vi "TCPIP_Server.vi"(9 "Message from Client":refnum<queue>, 10 "Data to TCPIP":refnum<queue>) -> ()   [LabVIEW 2018]
uses:
  TCP Multiple Connections State.ctl
  TCP Multiple Connections Data.ctl
panel:
  out "# of Connections":i32
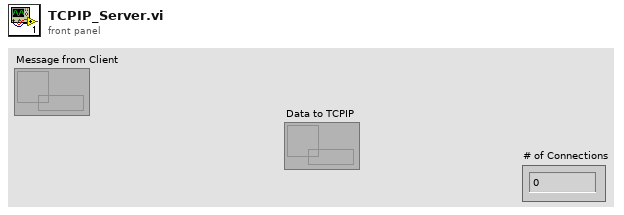
[diagram p1: front panel]
types:
  T1 = typedef "TCP Multiple Connections Data.ctl" = cluster{"Clients":refnum<k5>[], "Listener":refnum<k5>}
  T2 = typedef "TCP Multiple Connections State.ctl" = enum16{"Initialize", "Status Check", "Send Data", "Stop"}
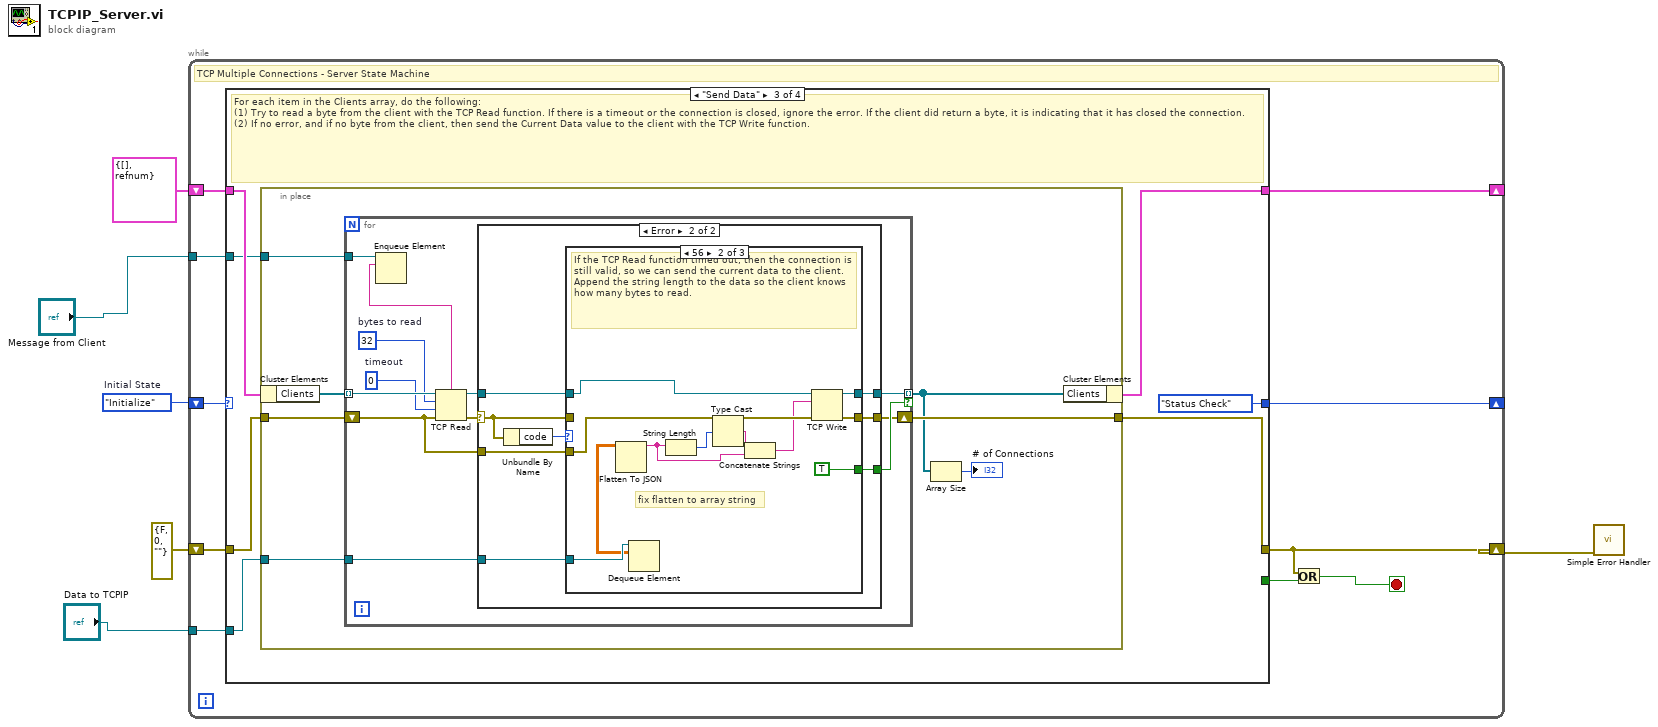
[diagram p0: block diagram]
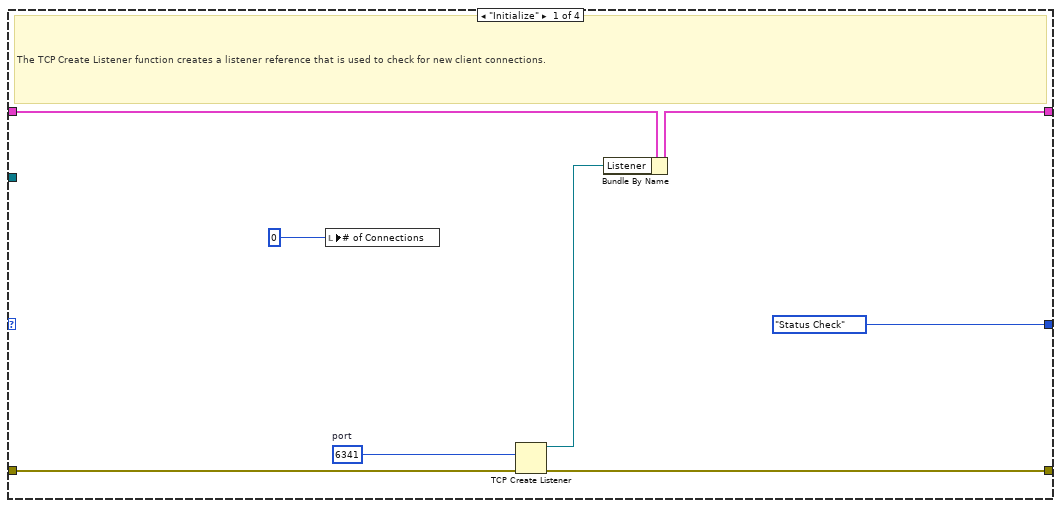
[diagram p2: hidden frame]
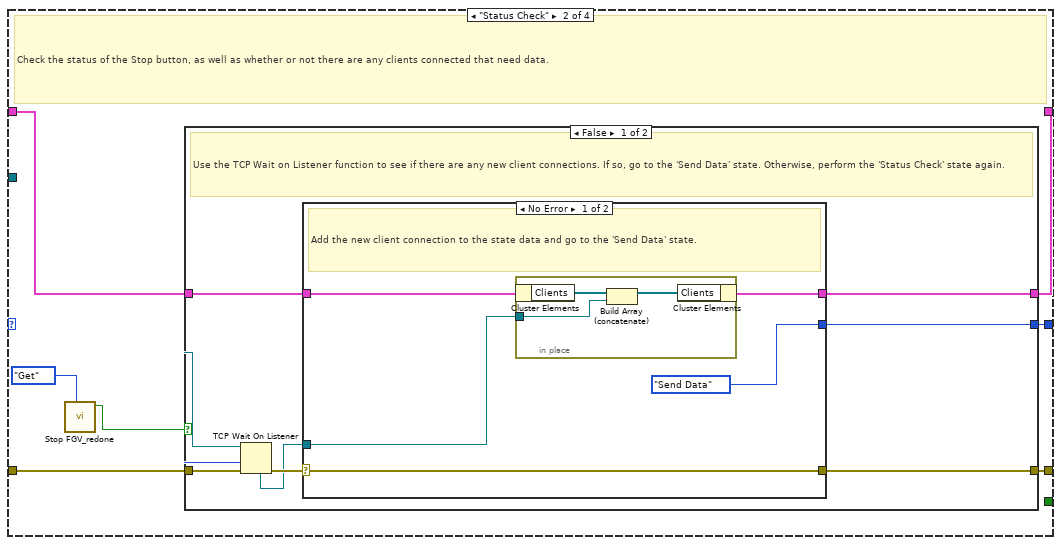
[diagram p3: hidden frame]
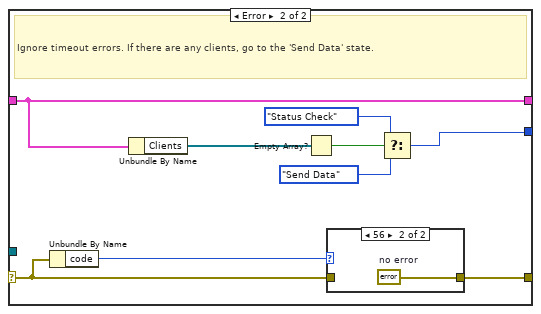
[diagram p4: hidden frame]
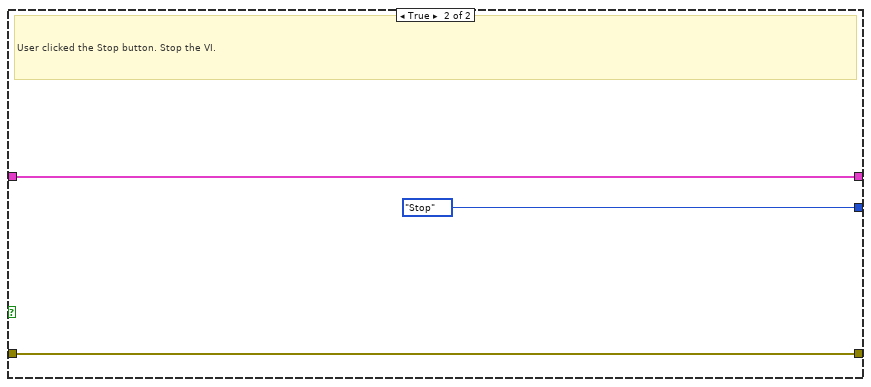
[diagram p6: hidden frame]
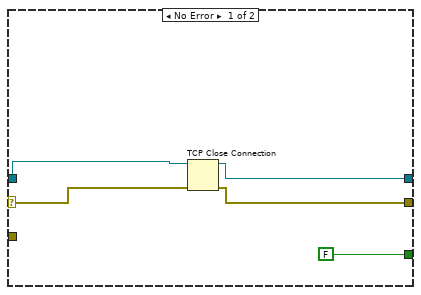
[diagram p7: hidden frame]
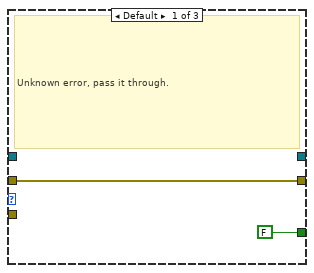
[diagram p8: hidden frame]
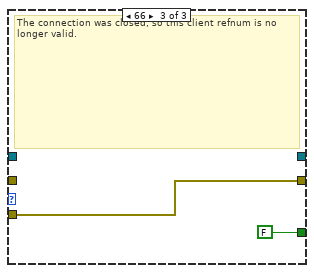
[diagram p9: hidden frame]
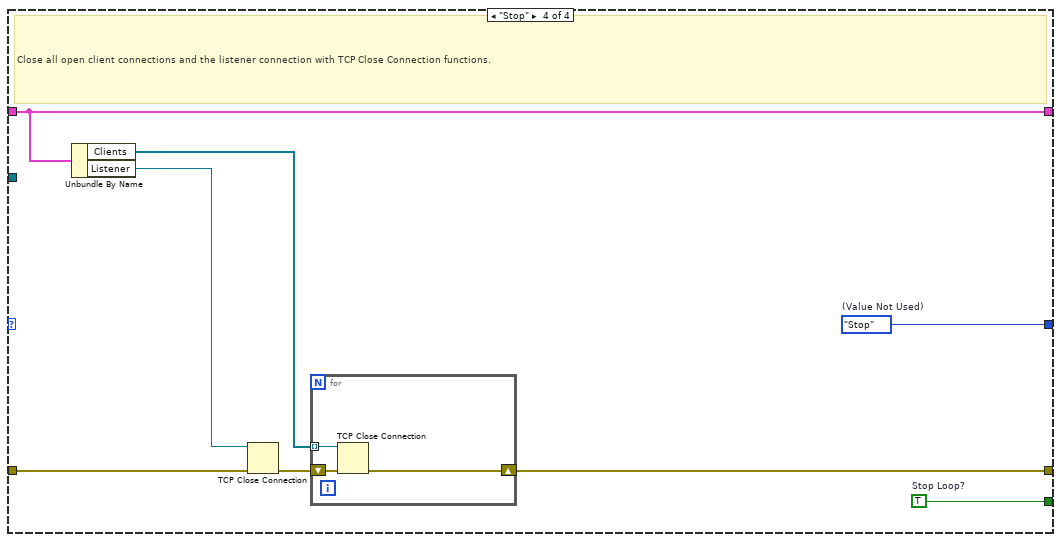
[diagram p10: hidden frame]
diagram:
  w6 = TCP_Multiple_Connections_State."Initialize"  # Initial State
  n1 = while {
    shift-right: [w15] -> _
    shift-left: w6 -> [w16]
    shift-right: [w13] -> _
    shift-left: T1 {"Clients"=[], "Listener"=refnum} ("Data") -> [w14]
    shift-right: [w9] -> w3
    shift-left: errorcluster {"status"=FALSE, "code"=0, "source"=""} ("error constant") -> [w12]
    tunnel: "Data to TCPIP" -> [w8]
    tunnel: "Message from Client" -> [w7]
    stop <- w10 stop-if-true
    # "TCP Multiple Connections - Server State Machine"
    n2 = case shown="\"Send Data\"" w16 {
      tunnel: [TCP_Multiple_Connections_State."Status Check" ("States") w31 TCP_Multiple_Connections_State."Status Check" ("States") w117] -> w15
      tunnel: [_ _ _ w124] -> w11
      tunnel: w14 -> [w22 w28 w67 w123]
      tunnel: [w21 w27 w66 w123] -> w13
      tunnel: w12 -> [w24 w30 w69 w122]
      tunnel: [w23 w29 w68 w120] -> w9
      tunnel: w8 -> [_ _ w64 _]
      tunnel: w7 -> [_ _ w63 _]
      frame "Initialize" {
        w19 = u16 6341  # port
        # "The TCP Create Listener function creates a listener reference that is used to check for new client connections."
        n3 = local write "# of Connections"(0 ("Number of Client Connections")) -> ()
        n4 = TCP Create Listener(8:w24, 10:w19) -> (0:w23:errorcluster, 3:w20:refnum<k5>)  [unwired: 4 out]
        n5 = Bundle By Name(cluster=w22, "Listener"=w20) -> (w21:T1)
      }
      frame "Status Check" {
        # "Check the status of the Stop button, as well as whether or not there are any clients connected that need data."
        n6 = call "Stop FGV_redone.vi"("Mode"=enum16{"Set", "Get"}."Get") -> ("Get Value"=w25:bool)  [unwired: 9 in, 1 out]
        n7 = case shown="False" w25 {
          tunnel: [w40 TCP_Multiple_Connections_State."Stop" ("States")] -> w31
          tunnel: w30 -> [w39 w62]
          tunnel: [w32 w62] -> w29
          tunnel: w28 -> [w35 w61]
          tunnel: [w34 w61] -> w27
          frame False {
            w38 = 100  # timeout ms
            # "Use the TCP Wait on Listener function to see if there are any new client connections. If so, go to the 'Send Data' state. Otherwise, perform the 'Status Check' state again."
            n8 = Unbundle By Name(w35) -> ("Listener"=w33:refnum<k5>)
            n9 = TCP Wait On Listener(8:w39, 9:w38, 11:w33) -> (0:w37:errorcluster, 4:w36:refnum<k5>)  [unwired: 4 out]
            n10 = case shown="No Error" w37 {
              selector: w37 -> [w43 w57]
              tunnel: [TCP_Multiple_Connections_State."Send Data" ("States") w51] -> w40
              tunnel: w36 -> [w44 _]
              tunnel: w35 -> [w45 w54]
              tunnel: [w42 w54] -> w34
              tunnel: [w43 w55] -> w32
              frame No Error {
                # "Add the new client connection to the state data and go to the 'Send Data' state."
                n11 = in-place {
                  in-place-border: w44 -> [w46]
                  n12 = in-place-cluster #1(w45) -> ("Clients"=w48:refnum<k5>[])
                  n13 = Build Array (concatenate)(w48, w46) -> (w47:refnum<k5>[])
                  n14 = in-place-cluster #1("Clients"=w47) -> (w42:T1)
                }
              }
              frame Error {
                # "Ignore timeout errors. If there are any clients, go to the 'Send Data' state."
                n15 = Unbundle By Name(w57) -> ("code"=w56:i32)
                n16 = Unbundle By Name(w54) -> ("Clients"=w53:refnum<k5>[])
                n17 = Empty Array?(array=w53) -> (empty?=w52:bool)
                n18 = case shown="56" w56 {
                  tunnel: w57 -> [w58 _]
                  tunnel: [w58 w59] -> w55
                  frame Default {
                  }
                  frame 56 {
                    w59 = errorcluster {"status"=FALSE, "code"=0, "source"=""}  # no error
                  }
                }
                n19 = Select(t=TCP_Multiple_Connections_State."Status Check" ("States"), s=w52, f=TCP_Multiple_Connections_State."Send Data" ("States")) -> (s? t:f=w51:T2)
              }
            }
          }
          frame True {
            # "User clicked the Stop button. Stop the VI."
          }
        }
      }
      frame "Send Data" {
        # "For each item in the Clients array, do the following:\n(1) Try to read a byte from the client with the TCP Read function. If there is a timeout or the connection is closed, ignore the error. If the client did return a byte, it is indicating that it has closed the connection.\n(2) If no error, and if no byte from the client, then send the Current Data value to the client with the TCP Write function."
        n20 = in-place {
          in-place-border: w69 -> [w76]
          in-place-border: [w75] -> w68
          in-place-border: w64 -> [w71]
          in-place-border: w63 -> [w70]
          n21 = in-place-cluster #2(w67) -> ("Clients"=w73:refnum<k5>[])
          n22 = for {
            tunnel: w73 -> [w88] mode=indexing
            shift-right: [w81] -> w75
            shift-left: w76 -> [w80]
            tunnel: [w83] -> w72 mode=indexing if=w82
            tunnel: w71 -> [w79]
            tunnel: w70 -> [w78]
            w85 = 0  # timeout
            w86 = 32  # bytes to read
            n23 = TCP Read(connection ID=w88, bytes to read=w86, error in (no error)=w80, 9:w85) -> (connection ID out=w87:refnum<k5>, data out=w77:string, error out=w84:errorcluster)  [unwired: 1 out]
            n24 = Enqueue Element(queue=w78, element=w77) -> ()  [unwired: 2 in, 3 out]
            n25 = case shown="Error" w84 {
              selector: w84 -> [w91 w100]
              tunnel: w87 -> [w92 w97]
              tunnel: [w90 w95] -> w83
              tunnel: [FALSE w96] -> w82
              tunnel: [w89 w99] -> w81
              tunnel: w80 -> [_ w98]
              tunnel: w79 -> [_ w94]
              frame No Error {
                # "If the client sent data, it is saying that the connection should be closed."
                n26 = TCP Close Connection(connection ID=w92, error in (no error)=w91) -> (connection ID out=w90:refnum<k5>, error out=w89:errorcluster)  [unwired: 1 in]
              }
              frame Error {
                # "Ignore connection closed and timeout errors"
                n27 = Unbundle By Name(w100) -> ("code"=w101:i32)
                n28 = case shown="56" w101 {
                  tunnel: w100 -> [w103 _ _]
                  tunnel: [w103 w114 w116] -> w99
                  tunnel: w98 -> [_ w111 w116]
                  tunnel: w97 -> [_ w108 _]
                  tunnel: [FALSE TRUE FALSE] -> w96
                  tunnel: [_ w113 _] -> w95
                  tunnel: w94 -> [_ w107 _]
                  frame Default {
                    # "Unknown error, pass it through."
                  }
                  frame 56 {
                    # "fix flatten to array string"
                    # "If the TCP Read function timed out, then the connection is still valid, so we can send the current data to the client. Append the string length to the data so the client knows how many bytes to read."
                    n29 = Dequeue Element(queue=w107) -> (element=w105:dbl[][])  [unwired: 2 in, 3 out]
                    n30 = Flatten To JSON(anything=w105) -> (JSON string=w104:string)  [unwired: 2 in, 1 out]
                    n31 = String Length(string=w104) -> (length=w106:i32)
                    n32 = Type Cast(x=w106) -> (*(type *) &x=w110:string)  [unwired: 1 in]
                    n33 = Concatenate Strings(w110, w104) -> (w109:string)
                    n34 = TCP Write(connection ID=w108, data in=w109, error in (no error)=w111) -> (connection ID out=w113:refnum<k5>, error out=w114:errorcluster)  [unwired: 2 out]
                  }
                  frame 66 {
                    # "The connection was closed, so this client refnum is no longer valid."
                  }
                }
              }
            }
          }
          n35 = Array Size(array=w72) -> (size(s)=→"# of Connections":i32)
          n36 = in-place-cluster #2("Clients"=w72) -> (w66:T1)
        }
      }
      frame "Stop" {
        w117 = TCP_Multiple_Connections_State."Stop"  # (Value Not Used)
        w124 = TRUE  # Stop Loop?
        # "Close all open client connections and the listener connection with TCP Close Connection functions."
        n37 = Unbundle By Name(w123) -> ("Clients"=w121:refnum<k5>[], "Listener"=w118:refnum<k5>)
        n38 = TCP Close Connection(connection ID=w118, error in (no error)=w122) -> (error out=w119:errorcluster)  [unwired: 1 in, 1 out]
        n39 = for {
          shift-right: [w126] -> w120
          shift-left: w119 -> [w127]
          tunnel: w121 -> [w125] mode=indexing
          n40 = TCP Close Connection(connection ID=w125, error in (no error)=w127) -> (error out=w126:errorcluster)  [unwired: 1 in, 1 out]
        }
      }
    }
    n41 = Or(x=w9, y=w11) -> (x .or. y?=w10:bool)
  }
  n42 = call <vilib>:"Simple Error Handler.vi"("error in (no error)"=w3) -> ()  [unwired: 4 in, 5 out]
